vi "JSON_Find_PARAM.vi"(8 "error in (no error)":errorcluster, 10 "data":string, 11 "name":string) -> (0 "error out":errorcluster, 3 "String":string)   [LabVIEW 2018]
uses:
  <vilib>/addons/JSON API/JSON Value/JSON Value.lvclass
  <vilib>/addons/JSON API/JSON Value/Get Item by name array.vi
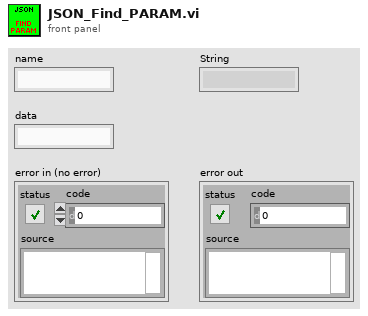
[diagram p1: front panel]
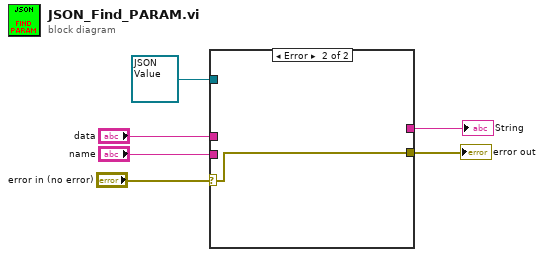
[diagram p0: block diagram]
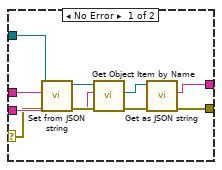
[diagram p2: hidden frame]
diagram:
  n1 = case shown="Error" "error in (no error)" {
    selector: "error in (no error)" -> [w7 w17]
    tunnel: refnum<class "JSON Value.lvclass"> refnum ("JSON Value In") -> [w16 _]
    tunnel: "data" -> [w11 _]
    tunnel: [w8 _] -> w5
    tunnel: [w9 w17] -> w6
    tunnel: "name" -> [w10 _]
    frame No Error {
      n2 = call <vilib>:"Set from JSON string.vi"("error in (no error)"=w7, "JSON stream"=w11, "JSON Value in"=w16) -> ("error out"=w13:errorcluster, "JSON Value out"=w12:refnum<class "JSON Value.lvclass">)  [unwired: 6 in, 1 out]
      n3 = call <vilib>:"Get Object Item by Name.vi"("error in (no error)"=w13, "name"=w10, "JSON Value In"=w12) -> ("error out"=w14:errorcluster, "Value"=w15:refnum<class "JSON Value.lvclass">)  [unwired: 5 in, 2 out]
      n4 = call <vilib>:"Get as JSON string.vi"("error in (no error)"=w14, "JSON Value in"=w15) -> ("error out"=w9:errorcluster, "<JSON>"=w8:string)  [unwired: 8 in]
    }
    frame Error {
    }
  }
  "error out" <- w6
  "String" <- w5
